vi "MCL Read Wave Form N.vi"(6 "handle":i32, 7 "waveform":dbl, 8 "error in (no error)":errorcluster, 9 "milliseconds":dbl, 10 "DataPoints":u32, 11 "axis":u32) -> (0 "error out":errorcluster, 3 "function return":i32, 5 "waveform out":dbl)   [LabVIEW 2014, in "Madlib.lvlib"]
doc: "MADLIB_API int MCL_ReadWaveFormN(unsigned int axis,unsigned int DataPoints,double milliseconds,double* waveform, int handle);"
uses:
  Madlib.lvlib
  Madlib.dll
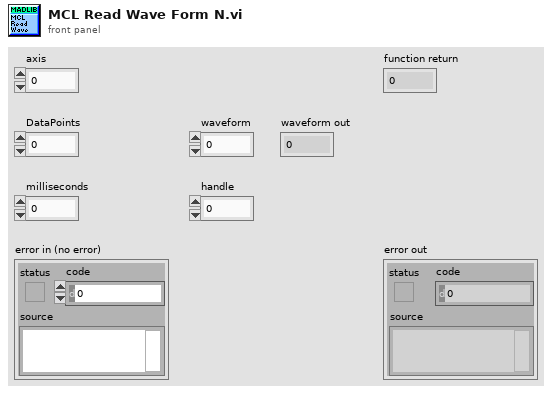
[diagram p1: front panel]
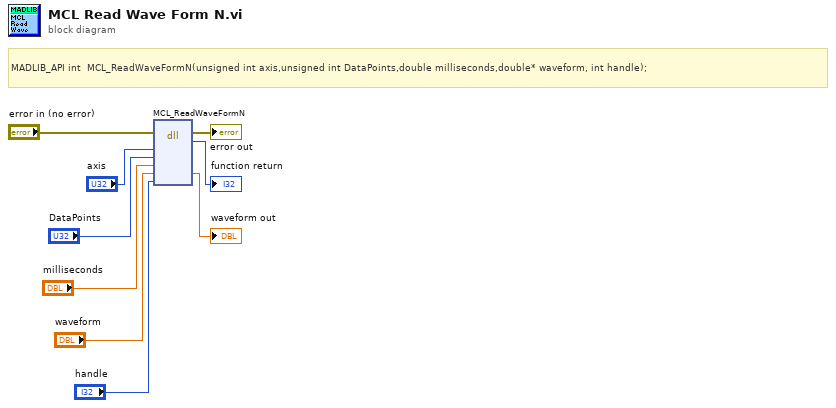
[diagram p0: block diagram]
diagram:
  # "MADLIB_API\tint\t\tMCL_ReadWaveFormN(unsigned int axis,unsigned int DataPoints,double milliseconds,double* waveform, int handle);"
  n1 = dll-call lib="C:/Users/Bakir/Desktop/LabFiles/TIRF-Microscope/Library Files - Andor and MadCity/Madlib/Madlib.*" fn="MCL_ReadWaveFormN"(error in="error in (no error)", "axis"="axis", "DataPoints"="DataPoints", "milliseconds"="milliseconds", "waveform"="waveform", "handle"="handle") -> (error out=→"error out":errorcluster, →"function return":i32, "waveform"=→"waveform out":dbl)  [unwired: 6 in, 1 out]
